vi "SelfTest.vi"(8 "error in (no error)":errorcluster, 11 "SpecAnBase in":refnum<class "SpecAnBase.lvclass">) -> (0 "error out":errorcluster, 1 "SelfTest Message":string, 2 "SelfTestResult":i16, 3 "SpecAnBase out":refnum<class "SpecAnBase.lvclass">)   [LabVIEW 2018, in "SpecAnPlugins.lvlib" / "SpecAnBase.lvclass"]
doc: "This VI runs the instrument's self test routine and returns the test result(s)."
uses:
  SpecAnBase.lvclass
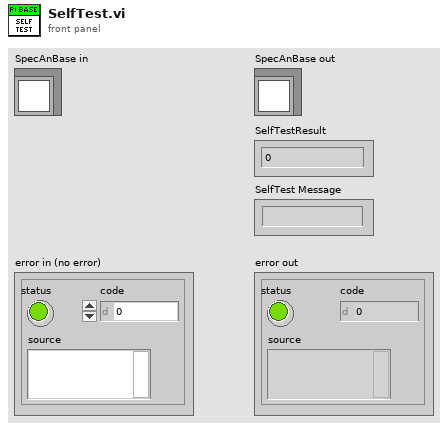
[diagram p1: front panel]
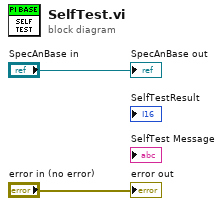
[diagram p0: block diagram]
diagram:
  "error out" <- "error in (no error)"
  "SpecAnBase out" <- "SpecAnBase in"
